vi "Get Installed Set.vi"(8 "error in (no error)":errorcluster, 9 "Cached (F)":bool, 10 "Item Types (all visible)":T1 items=["all visible", "all including hidden", "standard only", "startup only"], 11 "Session in":refnum<k21>) -> (0 "error out":errorcluster, 2 "Software Set":T2 {"information"."component type" items=["standard", "hidden", "system", "unknown", "startup", "image"]; "items"."component type" items=["standard", "hidden", "system", "unknown", "startup", "image"]; "add-ons"."component type" items=["standard", "hidden", "system", "unknown", "startup", "image"]}, 3 "Session out":refnum<k21>)   [LabVIEW 2014, in "nisyscfg.lvlib"]
doc: "Retrieves the software set installed on a Real-Time system. Not all systems support the installation of software sets."
uses:
  nisyscfg.lvlib
  Software Set 1.2.ctl
  Software 1.2.ctl
  Component Type.ctl
  Component Types.ctl
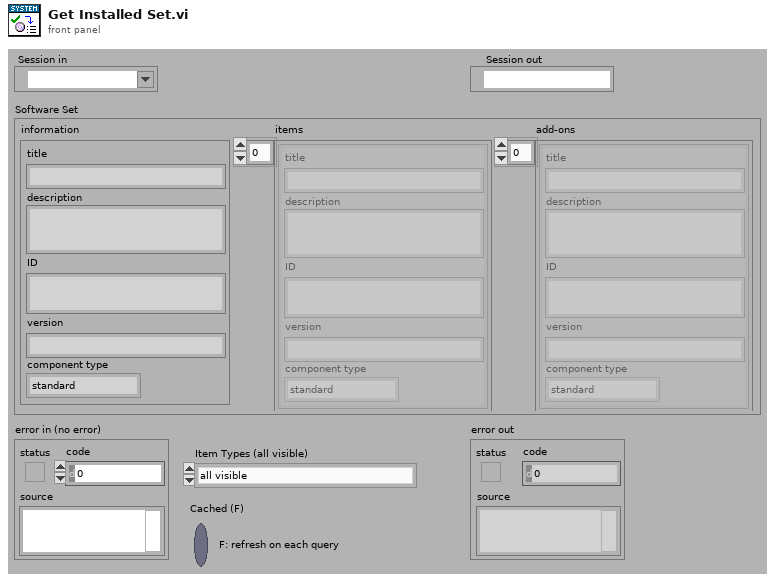
[diagram p1: front panel]
types:
  T1 = typedef "nisyscfg.lvlib/Component Types.ctl" = u32
  T2 = typedef "nisyscfg.lvlib/Software Set 1.2.ctl" = cluster{"information":T3, "items":T3[], "add-ons":T3[]}
  T3 = typedef "nisyscfg.lvlib/Software 1.2.ctl" = cluster{"title":string, "description":string, "ID":string, "version":string, "component type":T4}
  T4 = typedef "nisyscfg.lvlib/Component Type.ctl" = u32
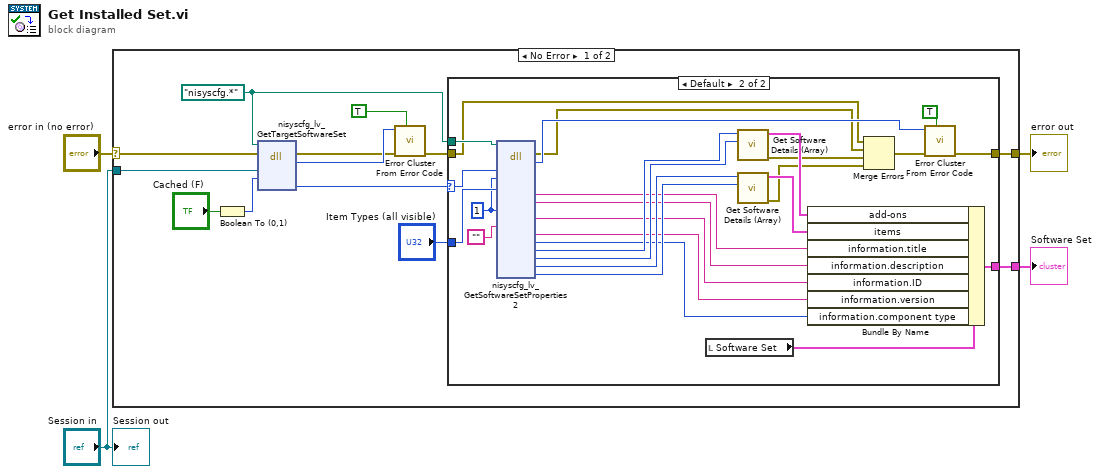
[diagram p0: block diagram]
diagram:
  n1 = case shown="No Error" "error in (no error)" {
    selector: "error in (no error)" -> [w12 w45]
    tunnel: [w14 w45] -> w4
    tunnel: [w13 _] -> w3
    tunnel: "Session in" -> [w11 _]
    frame No Error {
      w10 = path "nisyscfg.*" ("path in")
      n2 = Boolean To (0,1)(Boolean="Cached (F)") -> (0, 1=w7:i16)
      n3 = dll-call lib="nisyscfg.*" fn="nisyscfg_lv_GetTargetSoftwareSet" label="GetTargetSoftwareSet"(path in=w10, error in=w12, "session"=w11, "cached"=w7) -> (error out=w16:errorcluster, "result"=w17:i32, "softwareSet"=w6:u64)  [unwired: 4 in, 1 out]
      n4 = call "Error Cluster From Error Code.vi"("show call chain? (False)"=TRUE, "error in (no error)"=w16, "error code (0)"=w17) -> ("error out"=w15:errorcluster)  [unwired: 6 in]
      n5 = case shown="Default" w6 {
        selector: w6 -> [_ w36]
        tunnel: w15 -> [w18 w20]
        tunnel: [w18 w23] -> w14
        tunnel: [_ w43] -> w13
        tunnel: w10 -> [_ w42]
        tunnel: "Item Types (all visible)" -> [_ w28]
        frame 0 {
        }
        frame Default {
          w27 = u8 1 ("includeAddOnDeps")
          n6 = dll-call lib="nisyscfg.*" fn="nisyscfg_lv_GetSoftwareSetProperties2" label="GetSoftwareSetProperties"(path in=w42, "set"=w36, "includeAddOnDeps"=w27, "includeTypes"=w28, "type"=w27, "groupID"="") -> (error out=w21:errorcluster, "result"=w44:i32, "title"=w30:string, "description"=w31:string, "ID"=w29:string, "version"=w25:string, "visibleType"=w26:i32, "addons"=w39:u64, "numAddons"=w35:i32, "items"=w38:u64, "numItems"=w34:i32)  [unwired: 16 in, 1 out]
          n7 = local read "Software Set"() -> (w37:T2)
          n8 = call "Get Software Details (Array).vi"("Number of Elements"=w35, "Enumerator in"=w39) -> ("error out"=w22:errorcluster, "Software Components"=w32:T3[])  [unwired: 8 in]
          n9 = call "Get Software Details (Array).vi"("Number of Elements"=w34, "Enumerator in"=w38) -> ("error out"=w19:errorcluster, "Software Components"=w33:T3[])  [unwired: 8 in]
          n10 = Bundle By Name(cluster=w37, "add-ons"=w32, "items"=w33, "information.title"=w30, "information.description"=w31, "information.ID"=w29, "information.version"=w25, "information.component type"=w26) -> (w43:T2)
          n11 = Merge Errors(w20, w21, w22, w19) -> (w24:errorcluster)
          n12 = call "Error Cluster From Error Code.vi"("show call chain? (False)"=TRUE, "error in (no error)"=w24, "error code (0)"=w44) -> ("error out"=w23:errorcluster)  [unwired: 6 in]
        }
      }
    }
    frame Error {
    }
  }
  "error out" <- w4
  "Software Set" <- w3
  "Session out" <- "Session in"
